vi "Template.vi"() -> ()   [LabVIEW 2021]
uses:
  _Template/_Template.lvlib
  _Template/Script/Script/Script.lvclass
panel:
  in  "Create":bool
  in  "Template":string(combo)
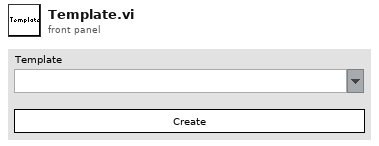
[diagram p1: front panel]
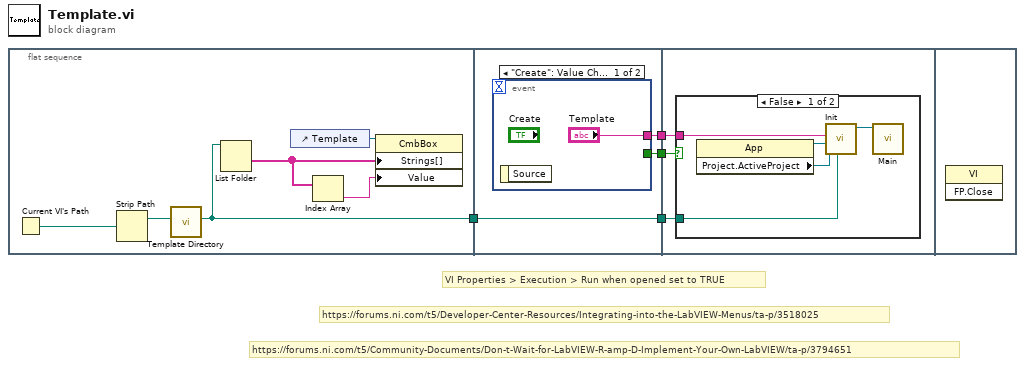
[diagram p0: block diagram]
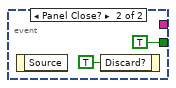
[diagram p2: hidden frame]
diagram:
  # "https://forums.ni.com/t5/Community-Documents/Don-t-Wait-for-LabVIEW-R-amp-D-Implement-Your-Own-LabVIEW/ta-p/3794651"
  # "https://forums.ni.com/t5/Developer-Center-Resources/Integrating-into-the-LabVIEW-Menus/ta-p/3518025"
  # "VI Properties > Execution > Run when opened set to TRUE"
  n1 = flat-sequence {
    tunnel: [w7] -> w4
    tunnel: w4 -> [w13]
    tunnel: [w13] -> w3
    tunnel: [w12] -> w2
    tunnel: [w11] -> w1
    tunnel: w3 -> [w19]
    tunnel: w2 -> [w18]
    tunnel: w1 -> [w17]
    frame #0 {
      n2 = Current VI's Path() -> (path=w9:path)
      n3 = Strip Path(path=w9) -> (stripped path=w8:path)  [unwired: 1 out]
      n4 = call "Template Directory.vi"("Base Path"=w8) -> ("Template Directory"=w7:path)  [unwired: 10 in]
      n5 = List Folder(path=w7) -> (folder names=w6:string[])  [unwired: 3 in, 3 out]
      n6 = control-ref of="Template"() -> (w10:refnum<vi>)
      n7 = Index Array(array=w6) -> (element=w5:string)  [unwired: 1 in]
      n8 = property class="CmbBox"(reference=w10, "Strings[]"=w6, "Value"=w5) -> ()  [unwired: 1 in, 2 out]
    }
    frame #1 {
      n9 = event shown="[0] \"Create\": Value Change" {
        selector: _ -> [_ _]
        dyn-events: _ -> [_ _]
        timeout: _ -> [_ _]
        tunnel: [_ TRUE] -> w12
        tunnel: ["Template" _] -> w11
        event "Create": Value Change {
          n10 = event-data() -> ()  [unwired: 1 in, 1 out]
        }
        event Panel Close? {
          n11 = event-data() -> ()  [unwired: 1 in, 1 out]
          n12 = event-data("Discard?"=TRUE) -> ()  [unwired: 1 in, 1 out]
        }
      }
    }
    frame #2 {
      n13 = case shown="False" w18 {
        tunnel: w17 -> [w21 _]
        tunnel: w19 -> [w20 _]
        frame False {
          n14 = property class="App"() -> (reference out=w24:refnum<vi>, "Project.ActiveProject"=w23:refnum<vi>)  [unwired: 2 in, 1 out]
          n15 = call "Init.vi"("Template Path"=w20, "Project:Active Project"=w23, "Application Instance"=w24, "Template Name"=w21) -> ("Script out"=w22:refnum<class "Script.lvclass">)  [unwired: 7 in]
          n16 = call "Main.vi"("Script in"=w22) -> ()  [unwired: 11 in]
        }
        frame True {
        }
      }
    }
    frame #3 {
      n17 = invoke class="VI" method="FP.Close"() -> ()  [unwired: 3 in, 3 out]
    }
  }
